vi "iWorx New Distance.vi"() -> ()   [LabVIEW 2012]
uses:
  <vilib>/DAQmx/write.llb/DAQmx Write (Analog Wfm 1Chan NSamp).vi
  <vilib>/DAQmx/read.llb/DAQmx Read (Analog Wfm 1Chan NSamp).vi
  <vilib>/DAQmx/create/channels.llb/DAQmx Create Channel (AI-Voltage-Basic).vi
  <vilib>/DAQmx/configure/timing.llb/DAQmx Timing (Sample Clock).vi
  <vilib>/DAQmx/create/channels.llb/DAQmx Create Channel (AO-Voltage-Basic).vi
  <vilib>/DAQmx/miscellaneous.llb/DAQmx Fill In Error Info.vi
  <vilib>/measure/mascope.llb/Pulse Measurements 1 chan.vi
  <vilib>/measure/NI_MABase.lvlib
  <vilib>/measure/NI_MAPro.lvlib
panel:
  out "error out":errorcluster
  out "Waveform Chart":dbl(graph)
  in  "Stop Button":bool
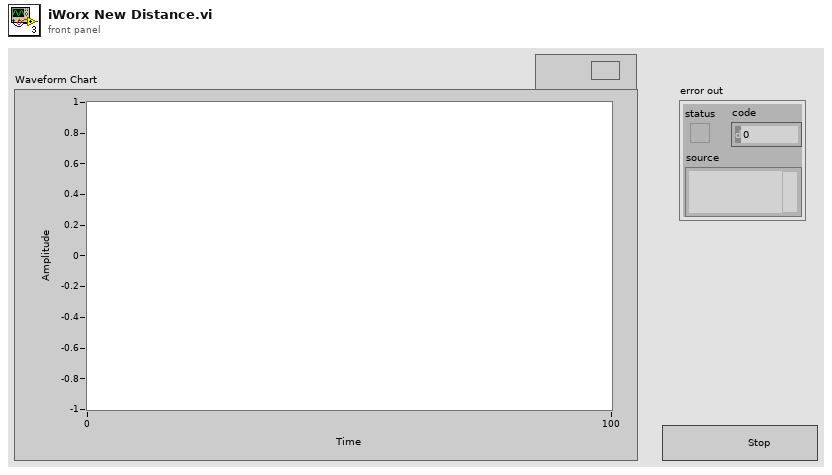
[diagram p1: front panel]
types:
  T1 = cluster{"high ref level":dbl, "mid ref level":dbl, "low ref level":dbl, "ref units":u16}
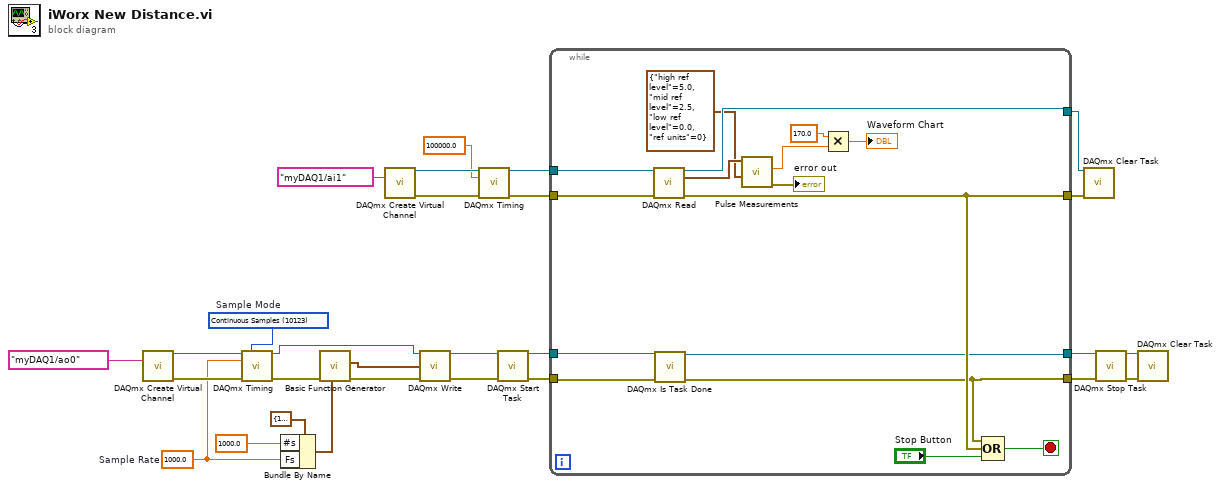
[diagram p0: block diagram]
diagram:
  w3 = 1000.0  # Sample Rate
  w20 = 10123 items=["Finite Samples"=10178, "Continuous Samples"=10123, "Hardware Timed Single Point"=12522]  # Sample Mode
  n1 = call-poly <vilib>:"DAQmx Create Virtual Channel.vi"("physical channels"=tag "myDAQ1/ao0" ("Physical Channel(s)")) -> ("task out"=w18:refnum<k21>, "error out"=w19:errorcluster)  [unwired: 13 in]
  n2 = call-poly <vilib>:"DAQmx Timing.vi"("task/channels in"=w18, "sample mode"=w20, "rate"=w3, "error in"=w19) -> ("task out"=w2:refnum<k21>, "error out"=w1:errorcluster)  [unwired: 10 in]
  n3 = Bundle By Name(cluster=cluster{"Fs":dbl, "#s":dbl} {"Fs"=1000.0, "#s"=1000.0} ("sampling info"), "#s"=1000.0 ("double precision float"), "Fs"=w3) -> (w15:cluster{"Fs":dbl, "#s":dbl})
  n4 = call <vilib>:"Basic Function Generator.vi"("sampling info"=w15, "error in (no error)"=w1) -> ("error out"=w12:errorcluster, "signal out"=w9:waveform(dbl))  [unwired: 7 in, 1 out]
  n5 = call-poly <vilib>:"DAQmx Create Virtual Channel.vi"("physical channels"=tag "myDAQ1/ai1") -> ("task out"=w27:refnum<k21>, "error out"=w26:errorcluster)  [unwired: 13 in]
  n6 = call-poly <vilib>:"DAQmx Write.vi"("task/channels in"=w2, "data"=w9, "error in"=w12) -> ("task out"=w14:refnum<k21>, "error out"=w13:errorcluster)  [unwired: 10 in, 1 out]
  n7 = call-poly <vilib>:"DAQmx Timing.vi"("task/channels in"=w27, "rate"=100000.0, "error in"=w26) -> ("task out"=w24:refnum<k21>, "error out"=w23:errorcluster)  [unwired: 11 in]
  n8 = call <vilib>:"DAQmx Start Task.vi"("task/channels in"=w14, "error in"=w13) -> ("task out"=w8:refnum<k21>, "error out"=w7:errorcluster)  [unwired: 12 in]
  n9 = while {
    tunnel: w8 -> [w32]
    tunnel: [w31] -> w6
    tunnel: w7 -> [w29]
    tunnel: [w30] -> w5
    tunnel: w24 -> [w42]
    tunnel: w23 -> [w41]
    tunnel: [w39] -> w22
    tunnel: [w38] -> w21
    stop <- w43 stop-if-true
    n10 = call-poly <vilib>:"DAQmx Read.vi"("task/channels in"=w42, "error in"=w41) -> ("task out"=w38:refnum<k21>, "data"=w40:waveform(dbl), "error out"=w39:errorcluster)  [unwired: 11 in]
    n11 = call <vilib>:"DAQmx Is Task Done.vi"("task/channels in"=w32, "error in"=w29) -> ("task out"=w31:refnum<k21>, "error out"=w30:errorcluster)  [unwired: 11 in, 1 out]
    n12 = call-poly <vilib>:"Pulse Measurements.vi"("reference levels"=T1 {"high ref level"=5.0, "mid ref level"=2.5, "low ref level"=0.0, "ref units"=0}, "signal in"=w40) -> ("error out"=→"error out":errorcluster, "pulse duration"=w37:dbl)  [unwired: 5 in, 3 out]
    n13 = Multiply(x=170.0, y=w37) -> (x*y=→"Waveform Chart":dbl)
    n14 = Compound Arithmetic op=OR(w30, w39, "Stop Button") -> (w43:bool)
  }
  n15 = call <vilib>:"DAQmx Clear Task.vi"("task in"=w21, "error in"=w22) -> ()  [unwired: 13 in, 1 out]
  n16 = call <vilib>:"DAQmx Stop Task.vi"("task/channels in"=w6, "error in"=w5) -> ("task out"=w11:refnum<k21>, "error out"=w10:errorcluster)  [unwired: 12 in]
  n17 = call <vilib>:"DAQmx Clear Task.vi"("task in"=w11, "error in"=w10) -> ()  [unwired: 13 in, 1 out]
